vi "R3 Time SBR Cycle.vi"(10 "Pump Status Array":bool[][](array[boolean])=[[TRUE, FALSE, TRUE, FALSE, FALSE], [TRUE, FALSE, FALSE, FALSE, TRUE], [FALSE, FALSE, FALSE, TRUE, FALSE], [FALSE, FALSE, FALSE, FALSE, FALSE], [FALSE, TRUE, FALSE, FALSE, FALSE], [FALSE, FALSE, FALSE, FALSE, FALSE]], 11 "Timing Array":u32[](array[numeric])=[80, 0, 25, 60, 5]) -> ()   [LabVIEW 2016]
uses:
  R3 Pump Manual Control.ctl
  R3Variables.lvlib
panel:
  in  "stop":bool
  out "Phase":dbl
  # "Call from Control.vi"
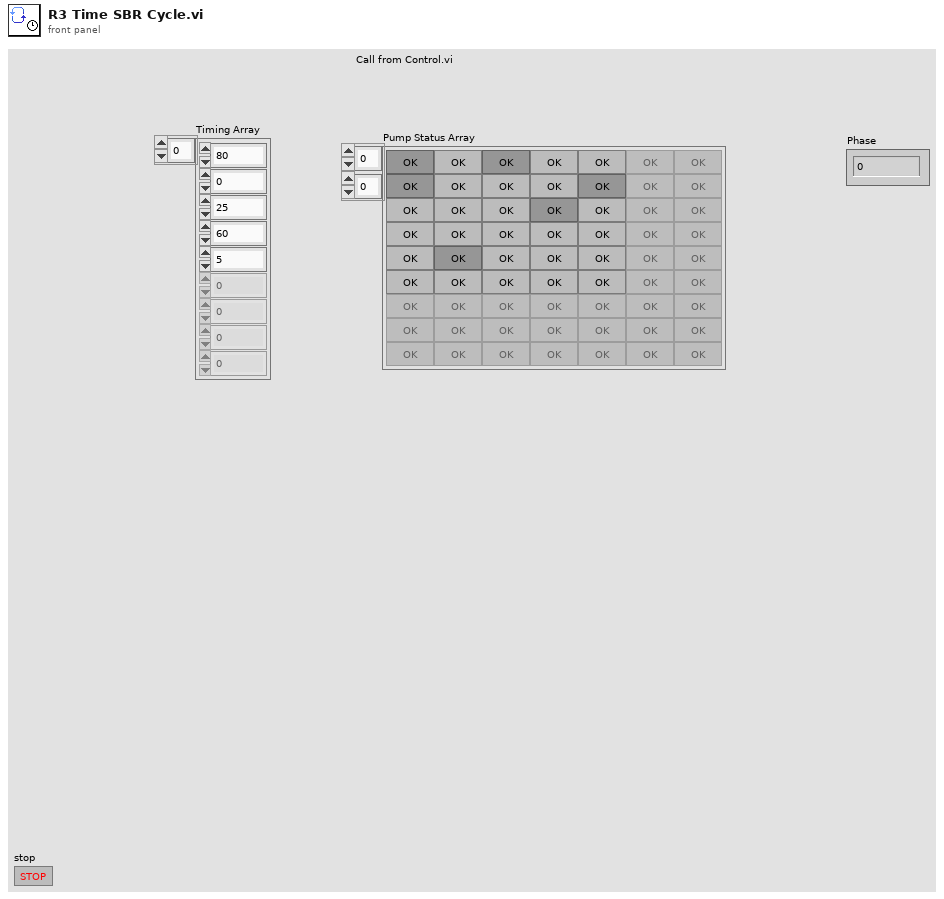
[diagram p1: front panel]
types:
  T1 = typedef "R3Variables.lvlib/R3 Pump Manual Control.ctl" = cluster{"AR Influent":bool, "AR Effluent":bool, "PR Feed":bool, "PR Decant":bool, "PR Recycle":bool, "PR Aeration":bool, "Stirring":bool}
  T2 = cluster{"Pump Status Array[0]":bool, "Pump Status Array[1]":bool, "Pump Status Array[2]":bool, "Pump Status Array[3]":bool, "Pump Status Array[4]":bool, "Pump Status Array[5]":bool, "Pump Status Array[6]":bool, "Pump Status Array[7]":bool, "Pump Status Array[8]":bool}
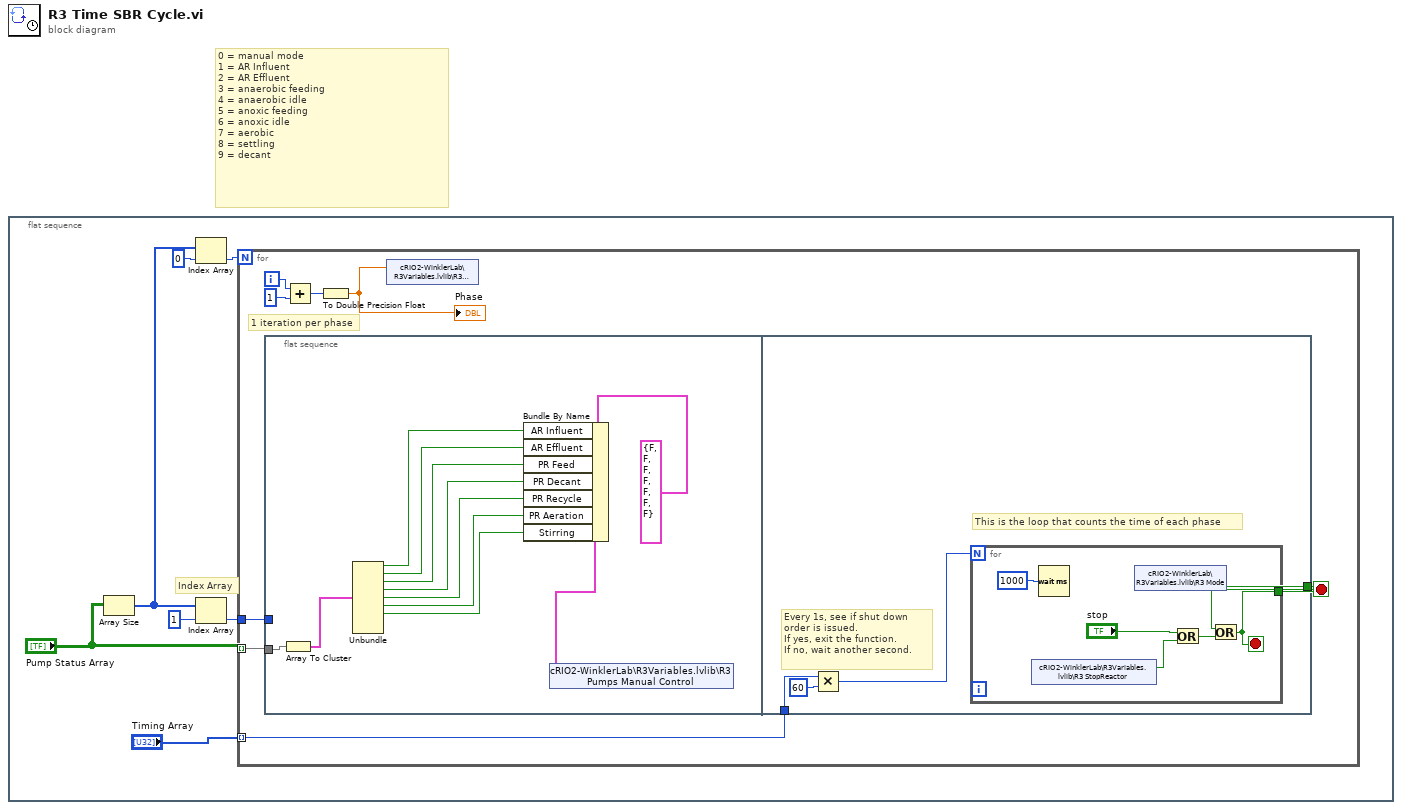
[diagram p0: block diagram]
diagram:
  # "0 = manual mode\n1 = AR Influent\n2 = AR Effluent\n3 = anaerobic feeding\n4 = anaerobic idle\n5 = anoxic feeding\n6 = anoxic idle\n7 = aerobic\n8 = settling\n9 = decant"
  n1 = flat-sequence {
    frame #0 {
      # "Index Array"
      n2 = Array Size(array="Pump Status Array") -> (size(s)=w5:i32[])
      n3 = Index Array(array=w5, index=0) -> (element=w2:i32)
      n4 = Index Array(array=w5, index=1) -> (element=w6:i32)
      n5 = for {
        N: w2 -> [_]
        tunnel: "Timing Array" -> [w13] mode=indexing
        tunnel: w6 -> [w15]
        tunnel: "Pump Status Array" -> [w14] mode=indexing
        i -> [w12]
        stop <- w8 stop-if-true
        # "1 iteration per phase"
        n6 = flat-sequence {
          tunnel: w15 -> [_]
          tunnel: w14 -> [w26]
          tunnel: w13 -> [w29]
          tunnel: [w28] -> w8
          frame #0 {
            n7 = Array To Cluster(array=w26) -> (cluster=w25:T2)
            n8 = Unbundle(w25) -> ("Pump Status Array[0]"=w23:bool, "Pump Status Array[1]"=w22:bool, "Pump Status Array[2]"=w21:bool, "Pump Status Array[3]"=w20:bool, "Pump Status Array[4]"=w19:bool, "Pump Status Array[5]"=w18:bool, "Pump Status Array[6]"=w17:bool)  [unwired: 2 out]
            n9 = Bundle By Name(cluster=T1 {"AR Influent"=FALSE, "AR Effluent"=FALSE, "PR Feed"=FALSE, "PR Decant"=FALSE, "PR Recycle"=FALSE, "PR Aeration"=FALSE, "Stirring"=FALSE} ("R3 Pumps Manual Control"), "AR Influent"=w23, "AR Effluent"=w22, "PR Feed"=w21, "PR Decant"=w20, "PR Recycle"=w19, "PR Aeration"=w18, "Stirring"=w17) -> (w24:T1)
            n10 = shared-variable "cRIO2-WinklerLab\\R3Variables.lvlib\\R3 Pumps Manual Control"(w24) -> ()  [unwired: 1 in, 1 out]
          }
          frame #1 {
            # "This is the loop that counts the time of each phase"
            # "Every 1s, see if shut down order is issued.\nIf yes, exit the function.\nIf no, wait another second."
            n11 = Multiply(x=w29, y=u32 60) -> (x*y=w27:u32)
            n12 = for {
              N: w27 -> [_]
              tunnel: [w32] -> w28
              stop <- w32 stop-if-true
              n13 = shared-variable "cRIO2-WinklerLab\\R3Variables.lvlib\\R3 StopReactor"() -> (w31:bool)  [unwired: 1 in, 1 out]
              n14 = Wait (ms)(milliseconds to wait=u32 1000) -> ()  [unwired: 1 out]
              n15 = shared-variable "cRIO2-WinklerLab\\R3Variables.lvlib\\R3 Mode"() -> (w33:bool)  [unwired: 1 in, 1 out]
              n16 = Or(x="stop", y=w31) -> (x .or. y?=w34:bool)
              n17 = Or(x=w33, y=w34) -> (x .or. y?=w32:bool)
            }
          }
        }
        n18 = Add(x=w12, y=1) -> (x+y=w10:i32)
        n19 = To Double Precision Float(number=w10) -> (double precision float=w9:dbl)
        "Phase" <- w9
        n20 = shared-variable "cRIO2-WinklerLab\\R3Variables.lvlib\\R3 Phase"(w9) -> ()  [unwired: 1 in, 1 out]
      }
    }
  }
